vi "개별 쓰기.vi"() -> ()   [LabVIEW 2014]
uses:
  <vilib>/Instr/_visa.llb/VISA Configure Serial Port (Instr).vi
panel:
  in  "WSS":bool
  in  "요구 프레임 WSB":string="\u000500WSB07%DW00020A3233303032333030323330303233303032333030\u0004"
  in  "요구 프레임 WSS":string="\u000500WSS0107%DW00003031\u0004"
  out "에러 출력":errorcluster={"status"=FALSE, "code"=1073676294, "source"="XGB 통신.vi->개별 쓰기.vi 안에 VISA 읽기"}
  in  "parity (0:none)":enum16{"None", "Odd", "Even", "Mark", "Space"}(ring) caption="패리티(0:없음)"
  in  "data bits (8)":u16=8 caption="데이터 비트(8)" min=5 max=8 step=1
  out "read buffer":string
  in  "baud rate (9600)":u32=115200 caption="보 전송속도(9600)"
  in  "VISA resource name":refnum<visa-resource-name>="COM1" caption="VISA 리소스 이름"
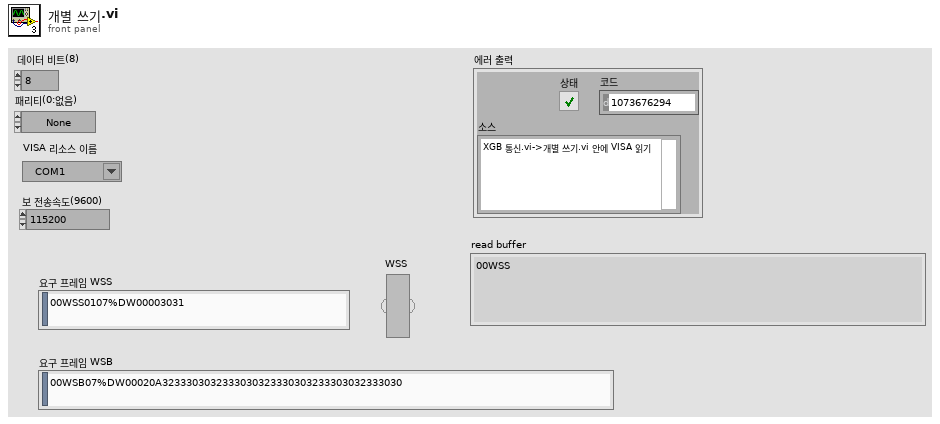
[diagram p1: front panel]
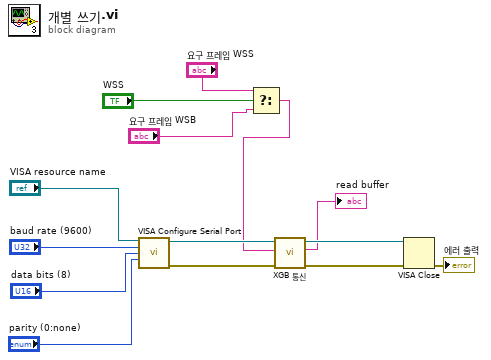
[diagram p0: block diagram]
diagram:
  n1 = call-poly "VISA Configure Serial Port"("VISA resource name"="VISA resource name", "baud rate (9600)"="baud rate (9600)", "data bits (8)"="data bits (8)", "parity (0:none)"="parity (0:none)") -> ("VISA resource name out"=w14:refnum<visa-resource-name>, "error out"=w12:errorcluster)  [unwired: 10 in]
  n2 = Select(t="요구 프레임 WSS", s="WSS", f="요구 프레임 WSB") -> (s? t:f=w1:string)
  n3 = call "XGB 통신.vi"("error in (no error)"=w12, "String"=w1, "VISA Refnum in"=w14) -> ("error out"=w5:errorcluster, "read buffer"=→"read buffer":string, "VISA Refnum out"=w13:refnum<visa-resource-name>)  [unwired: 5 in, 1 out]
  n4 = VISA Close(VISA resource name=w13, error in (no error)=w5) -> (error out=→"에러 출력":errorcluster)
